vi "UDP Send and Receive (repeat on error) - String.vi"(7 "timeout ms (100)":i32=100, 8 "error in (no error)":errorcluster, 9 "String Command & Param":T1, 10 "IP":string, 11 "connection ID in":refnum<k16>) -> (0 "error out":errorcluster, 2 "String Param out":string, 3 "connection ID out":refnum<k16>)   [LabVIEW 2016, in "SMD-7615.lvlib" / "eSCL.lvlib"]
doc: "AC - Acceleration Rate\nSets or requests the acceleration rate used in point-to-point move commands in rev/sec/sec."
uses:
  eSCL.lvlib
  String Command and Param.ctl
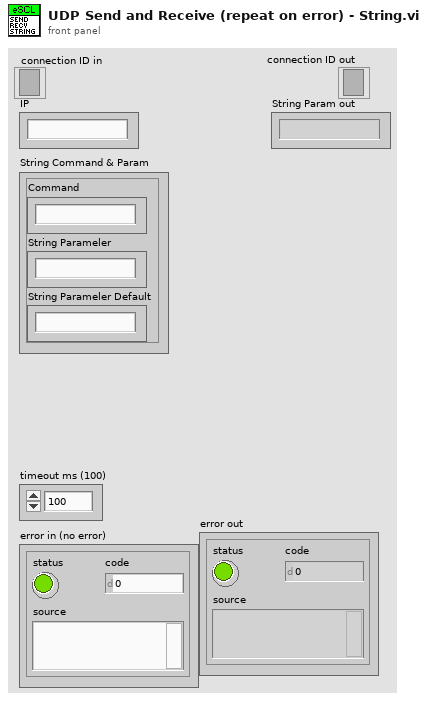
[diagram p1: front panel]
types:
  T1 = typedef "SMD-7615.lvlib/eSCL.lvlib/String Command and Param.ctl" = cluster{"Command":string, "String Parameler":string, "String Parameler Default":string}
  T2 = typedef "SMD-7615.lvlib/eSCL.lvlib/UDP Received Data.ctl" = cluster{"Received String":string, "eSCL Cmd":string, "Data":string}
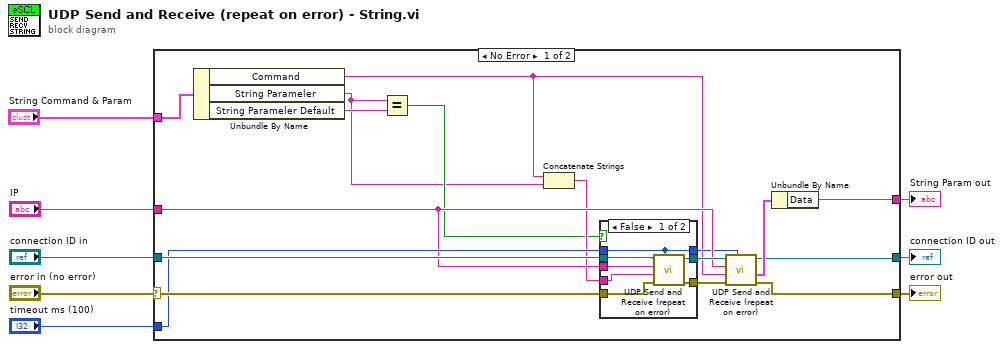
[diagram p0: block diagram]
diagram:
  n1 = case shown="No Error" "error in (no error)" {
    selector: "error in (no error)" -> [w25 w36]
    tunnel: "connection ID in" -> [w24 w37]
    tunnel: [w18 w37] -> w6
    tunnel: [w17 w36] -> w5
    tunnel: "IP" -> [w20 _]
    tunnel: "timeout ms (100)" -> [w21 _]
    tunnel: "String Command & Param" -> [w13 _]
    tunnel: [w9 _] -> w1
    frame No Error {
      n2 = Unbundle By Name(w13) -> ("Command"=w11:string, "String Parameler"=w10:string, "String Parameler Default"=w12:string)
      n3 = Equal?(x=w10, y=w12) -> (x = y?=w14:bool)
      n4 = Concatenate Strings(w11, w10) -> (w16:string)
      n5 = case shown="False" w14 {
        tunnel: w25 -> [w32 w33]
        tunnel: w24 -> [w31 w35]
        tunnel: [w30 w33] -> w23
        tunnel: [w29 w35] -> w22
        tunnel: w21 -> [w26 w34]
        tunnel: w20 -> [w28 _]
        tunnel: w16 -> [w27 _]
        tunnel: [w26 w34] -> w15
        frame False {
          n6 = call "UDP Send and Receive (repeat on error).vi"("timeout ms (100)"=w26, "error in (no error)"=w32, "Data"=w27, "IP"=w28, "connection ID in"=w31) -> ("error out"=w30:errorcluster, "connection ID out"=w29:refnum<k16>)  [unwired: 3 in, 2 out]
        }
        frame True {
        }
      }
      n7 = call "UDP Send and Receive (repeat on error).vi"("timeout ms (100)"=w15, "error in (no error)"=w23, "Data"=w11, "IP"=w20, "connection ID in"=w22) -> ("error out"=w17:errorcluster, "Received Data"=w19:T2, "connection ID out"=w18:refnum<k16>)  [unwired: 3 in, 1 out]
      n8 = Unbundle By Name(w19) -> ("Data"=w9:string)
    }
    frame Error {
    }
  }
  "connection ID out" <- w6
  "error out" <- w5
  "String Param out" <- w1
